vi "DownsampleStage_5761.vi"(8 "valid in":bool, 9 "reset":bool, 11 "Data in":fxp<+/-,16,14>[](array[numeric])=[0.0, 0.0, 0.0, 0.0, 0.0, 0.0, 0.0, 0.0]) -> (0 "valid out":bool, 3 "data out":fxp<+/-,16,14>[](array[numeric]))   [LabVIEW 2013]
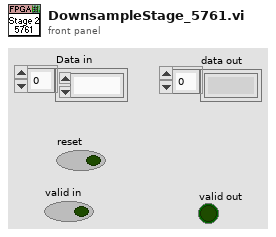
[diagram p1: front panel]
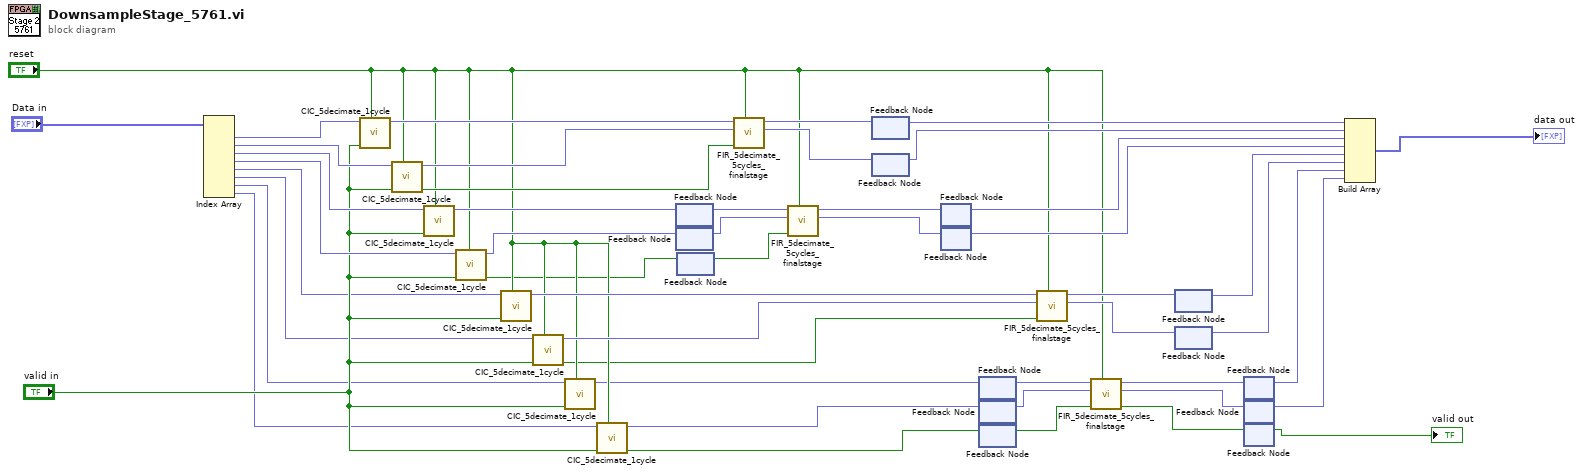
[diagram p0: block diagram]
diagram:
  n1 = Index Array(array="Data in") -> (element #1=w47:fxp<+/-,16,14>, element #2=w45:fxp<+/-,16,14>, element #3=w44:fxp<+/-,16,14>, element #4=w43:fxp<+/-,16,14>, element #5=w23:fxp<+/-,16,14>, element #6=w24:fxp<+/-,16,14>, element #7=w25:fxp<+/-,16,14>, element #8=w26:fxp<+/-,16,14>)  [unwired: 8 in]
  n2 = call "CIC_5decimate_1cycle.vi"("reset"="reset", "valid in"="valid in", "Data in"=w47) -> ("Data out"=w38:fxp<+/-,16,14>)  [unwired: 7 in, 1 out]
  n3 = call "CIC_5decimate_1cycle.vi"("reset"="reset", "valid in"="valid in", "Data in"=w45) -> ("valid out"=w36:bool, "Data out"=w37:fxp<+/-,16,14>)  [unwired: 7 in]
  n4 = call "CIC_5decimate_1cycle.vi"("reset"="reset", "valid in"="valid in", "Data in"=w44) -> ("Data out"=w42:fxp<+/-,16,14>)  [unwired: 7 in, 1 out]
  n5 = call "CIC_5decimate_1cycle.vi"("reset"="reset", "valid in"="valid in", "Data in"=w43) -> ("valid out"=w3:bool, "Data out"=w41:fxp<+/-,16,14>)  [unwired: 7 in]
  n6 = call "CIC_5decimate_1cycle.vi"("reset"="reset", "valid in"="valid in", "Data in"=w23) -> ("Data out"=w14:fxp<+/-,16,14>)  [unwired: 7 in, 1 out]
  n7 = call "CIC_5decimate_1cycle.vi"("reset"="reset", "valid in"="valid in", "Data in"=w24) -> ("valid out"=w1:bool, "Data out"=w13:fxp<+/-,16,14>)  [unwired: 7 in]
  n8 = call "CIC_5decimate_1cycle.vi"("reset"="reset", "valid in"="valid in", "Data in"=w25) -> ("Data out"=w11:fxp<+/-,16,14>)  [unwired: 7 in, 1 out]
  n9 = call "CIC_5decimate_1cycle.vi"("reset"="reset", "valid in"="valid in", "Data in"=w26) -> ("valid out"=w9:bool, "Data out"=w10:fxp<+/-,16,14>)  [unwired: 7 in]
  n10 = feedback #1() -> (w40:fxp<+/-,16,14>)  [unwired: 1 in]
  n11 = feedback-in #1(w42) -> ()
  n12 = feedback #2() -> (w39:fxp<+/-,16,14>)  [unwired: 1 in]
  n13 = feedback-in #2(w41) -> ()
  n14 = feedback #3() -> (w2:bool)  [unwired: 1 in]
  n15 = feedback-in #3(w3) -> ()
  n16 = call "FIR_5decimate_5cycles_finalstage.vi"("reset"="reset", "valid in"=w36, "Q in"=w37, "I in"=w38) -> ("Q out"=w34:fxp<+/-,16,14>, "I out"=w35:fxp<+/-,16,14>)  [unwired: 4 in, 2 out]
  n17 = call "FIR_5decimate_5cycles_finalstage.vi"("reset"="reset", "valid in"=w2, "Q in"=w39, "I in"=w40) -> ("Q out"=w30:fxp<+/-,16,14>, "I out"=w31:fxp<+/-,16,14>)  [unwired: 4 in, 2 out]
  n18 = feedback #4() -> (w33:fxp<+/-,16,14>)  [unwired: 1 in]
  n19 = feedback-in #4(w35) -> ()
  n20 = feedback #5() -> (w32:fxp<+/-,16,14>)  [unwired: 1 in]
  n21 = feedback-in #5(w34) -> ()
  n22 = feedback #6() -> (w28:fxp<+/-,16,14>)  [unwired: 1 in]
  n23 = feedback-in #6(w31) -> ()
  n24 = feedback #7() -> (w29:fxp<+/-,16,14>)  [unwired: 1 in]
  n25 = feedback-in #7(w30) -> ()
  n26 = feedback #8() -> (w15:fxp<+/-,16,14>)  [unwired: 1 in]
  n27 = feedback-in #8(w11) -> ()
  n28 = feedback #9() -> (w16:fxp<+/-,16,14>)  [unwired: 1 in]
  n29 = feedback-in #9(w10) -> ()
  n30 = feedback #10() -> (w17:bool)  [unwired: 1 in]
  n31 = feedback-in #10(w9) -> ()
  n32 = call "FIR_5decimate_5cycles_finalstage.vi"("reset"="reset", "valid in"=w1, "Q in"=w13, "I in"=w14) -> ("Q out"=w19:fxp<+/-,16,14>, "I out"=w18:fxp<+/-,16,14>)  [unwired: 4 in, 2 out]
  n33 = call "FIR_5decimate_5cycles_finalstage.vi"("reset"="reset", "valid in"=w17, "Q in"=w16, "I in"=w15) -> ("valid out"=w22:bool, "Q out"=w21:fxp<+/-,16,14>, "I out"=w20:fxp<+/-,16,14>)  [unwired: 4 in, 1 out]
  n34 = feedback #11() -> (w7:fxp<+/-,16,14>)  [unwired: 1 in]
  n35 = feedback-in #11(w18) -> ()
  n36 = feedback #12() -> (w6:fxp<+/-,16,14>)  [unwired: 1 in]
  n37 = feedback-in #12(w19) -> ()
  n38 = feedback #13() -> (w5:fxp<+/-,16,14>)  [unwired: 1 in]
  n39 = feedback-in #13(w20) -> ()
  n40 = feedback #14() -> (w4:fxp<+/-,16,14>)  [unwired: 1 in]
  n41 = feedback-in #14(w21) -> ()
  n42 = feedback #15() -> (→"valid out":bool)  [unwired: 1 in]
  n43 = feedback-in #15(w22) -> ()
  n44 = Build Array(w33, w32, w28, w29, w7, w6, w5, w4) -> (→"data out":fxp<+/-,16,14>[])
